vi "basement tank 2.vi"() -> ()   [LabVIEW 2019]
uses:
  <vilib>/NI/Current Value Table/Type Defs/Single Tag.ctl
  <vilib>/NI/Current Value Table/Type Defs/Data Types.ctl
  <vilib>/NI/STM/TCP/Read Meta Data (TCP Ref).vi
  <vilib>/NI/STM/TCP/Get Connection Reference (TCP).vi
  <vilib>/NI/AMC/Read Termination Message.vi
  <vilib>/NI/AMC/Create Single Message.vi
  <vilib>/NI/AMC/Update Message Routing Info.vi
  <vilib>/NI/STM/TCP/Read Meta Data (TCP Clst).vi
  <vilib>/NI/AMC/Globals.vi
  <vilib>/NI/STM/TCP/Write Message (TCP).vi
  <vilib>/NI/AMC/Send Message.vi
  <vilib>/NI/AMC/AMC.lvlib
  <vilib>/NI/STM/NI STM.lvlib
  <vilib>/NI/Current Value Table/Current Value Table.lvlib
panel:
  in  "Auto Level Main Tank":dbl(knob)=250.0 min=250.0 max=950.0 step=1.0 scale=200.0..1000.0 scale format="%#.3g"
  in  "Enable DI Auto Top-up":bool
  in  "CuOAddAmount":dbl caption="CuO grams to add" min=-1000.0 max=1000.0 step=1.0
  out "Grams CuO to Add":dbl format="%.1f"
  in  "Dose Extra Oxide":bool
  in  "Sulfuric Proc 2":dbl=2.0 caption="ml Acid Proc 2" min=0.0 max=5000.0 step=1.0
  in  "Trig Sulfuric Proc2":bool caption="Trigger Dose"
  out "Flow":bool
  in  "LEV Proc 2":dbl=2.0 caption="ml Lev Proc 2" min=0.0 max=1000.0 step=1.0
  in  "Trig Level Proc 2":bool caption="Trigger Dose"
  in  "UCON Proc 2":dbl=2.0 caption="ml UCON Proc 2" min=0.0 max=1000.0 step=1.0
  in  "Trig UCON Proc 2":bool caption="Trigger Dose"
  in  "SPS Proc 2":dbl=2.0 caption="ml SPS Proc 2" min=0.0 max=1000.0 step=1.0
  in  "Trig SPS Proc 2":bool caption="Trigger Dose"
  in  "BasT2_L Last Hr":bool
  in  "FlowInd OxSys":dbl(slide) scale=0.0..15.0
  in  "Supply Pressure (kPa)":dbl(knob)=50.0 min=50.0 max=200.0 step=5.0 scale=50.0..200.0
  in  "BasT2_P Last Hr":bool
  in  "BasT2_Flow Last Hr":bool
  out "Boiler Water Facilities Valve":dbl(slide) scale=0.0..100.0
  out "Tempered Water Facilities Valve":dbl(slide) scale=0.0..100.0
  out "Chilled Water Facilities Valve":dbl(slide) scale=0.0..100.0
  out "Total Flow (when operated with plating tanks)":dbl(knob) scale=0.0..150.0
  out "To Plating Process 3 & 4":bool
  out "ThreewayLowerElbow":bool
  out "PipeToTank":bool
  out "Tnk1Tee 2":bool
  out "PipeToPump 2":bool
  out "BTnk1 SG":dbl format="%.3f"
  in  "Specific Gravity":dbl(knob)=1.0 min=1.0 max=1.25 step=0.0025 scale=1.0..1.25
  out "OxideToFilter":bool
  out "Oxide Pump":bool
  out "Boolean 4":bool
  out "OxideDose Indicate":bool
  in  "Flow rate To Oxide":dbl(knob) scale=2.0..10.0
  in  "Oxide Dosing Enable":bool
  out "Chilled Injection":u8(slide) scale=0.0..100.0
  out "Tempered Injection":dbl(slide) scale=0.0..100.0
  in  "BasT3_T Last Hr":bool
  in  "Enable T-Control":bool
  in  "Temperature Setpoint":dbl(knob) step=0.1 scale=12.0..30.0 scale format="%#.1g"
  out "Boiler Water Out":dbl(knob) scale=10.0..110.0
  out "Boiler Water In":dbl(knob) scale=10.0..110.0
  out "Tempered Water Out":dbl(knob) scale=10.0..35.0
  out "Tempered Water In":dbl(knob) scale=10.0..35.0
  out "Chilled Water Out":dbl(knob) scale=0.0..25.0
  out "Chilled Water In":dbl(knob) scale=0.0..25.0
  in  "Tab Control":enum32{"Main Pump", "Lift Pump"}(tab)
  out "Amps":dbl format="%#.2g"
  out "Volts":dbl format="%#.1f"
  out "VFD T":dbl format="%#.2g"
  out "RPM":dbl format="%#.2f"
  out "Fault Code":dbl format="%#.2g"
  out "Freq":dbl format="%#.2g"
  out "Fault Code Ox Pmp":dbl caption="Fault Code" format="%#.2g"
  out "VFD T Ox Pmp":dbl caption="VFD T" format="%#.2g"
  out "Amps Ox Pmp":dbl caption="Amps" format="%#.2g"
  out "Volts Ox Pmp":dbl caption="Volts" format="%#.1f"
  out "Boolean 6":bool
  out "Circulator":bool
  out "HeatExchanger":bool
  out "Main Pump":bool
  out "Supply Pressure (kPa)":dbl(knob) scale=0.0..250.0
  out "Total Added":dbl format="%.2g"
  out "DI Flow (L/min)":dbl(knob) scale=0.0..100.0
  in  "Liters DI to Add":dbl(knob) min=0.0 max=500.0 step=1.0 scale=0.0..500.0
  in  "Add DI Water":bool
  in  "Drain System to Tree":bool
  in  "Enable Main Pump":bool
  out "E Stop":bool
  out "Run Enabled?":bool
  out "Supply Temperature":dbl(slide) scale=0.0..100.0
  out "Tank":dbl(slide) scale=0.0..1000.0
  in  "Machine":bool
  in  "Basement 4":bool
  in  "Dryer":bool
  in  "Rinse 4":bool
  in  "Rinse 3":bool
  in  "Rinse 2":bool
  in  "Basement 3":bool
  in  "Basement 2":bool
  in  "Basement 1":bool
  in  "Plater 6":bool
  in  "Plater 5":bool
  in  "Plater 4":bool
  in  "Plater 3":bool
  in  "Plater 2":bool
  in  "Plater 1":bool
  in  "Predip":bool
  in  "Rinse 1":bool
  in  "Cleaner":bool
  in  "Etch":bool
  out "status":string
  out "Tnk1Tee":bool
  out "PipeToPump":bool
  # "Module Selection"
  # "@"
  # "SG"
  # "L/min"
  # "Dosing"
  # "SPS"
  # "UCON"
  # "Leveler"
  # "Sulfuric Acid"
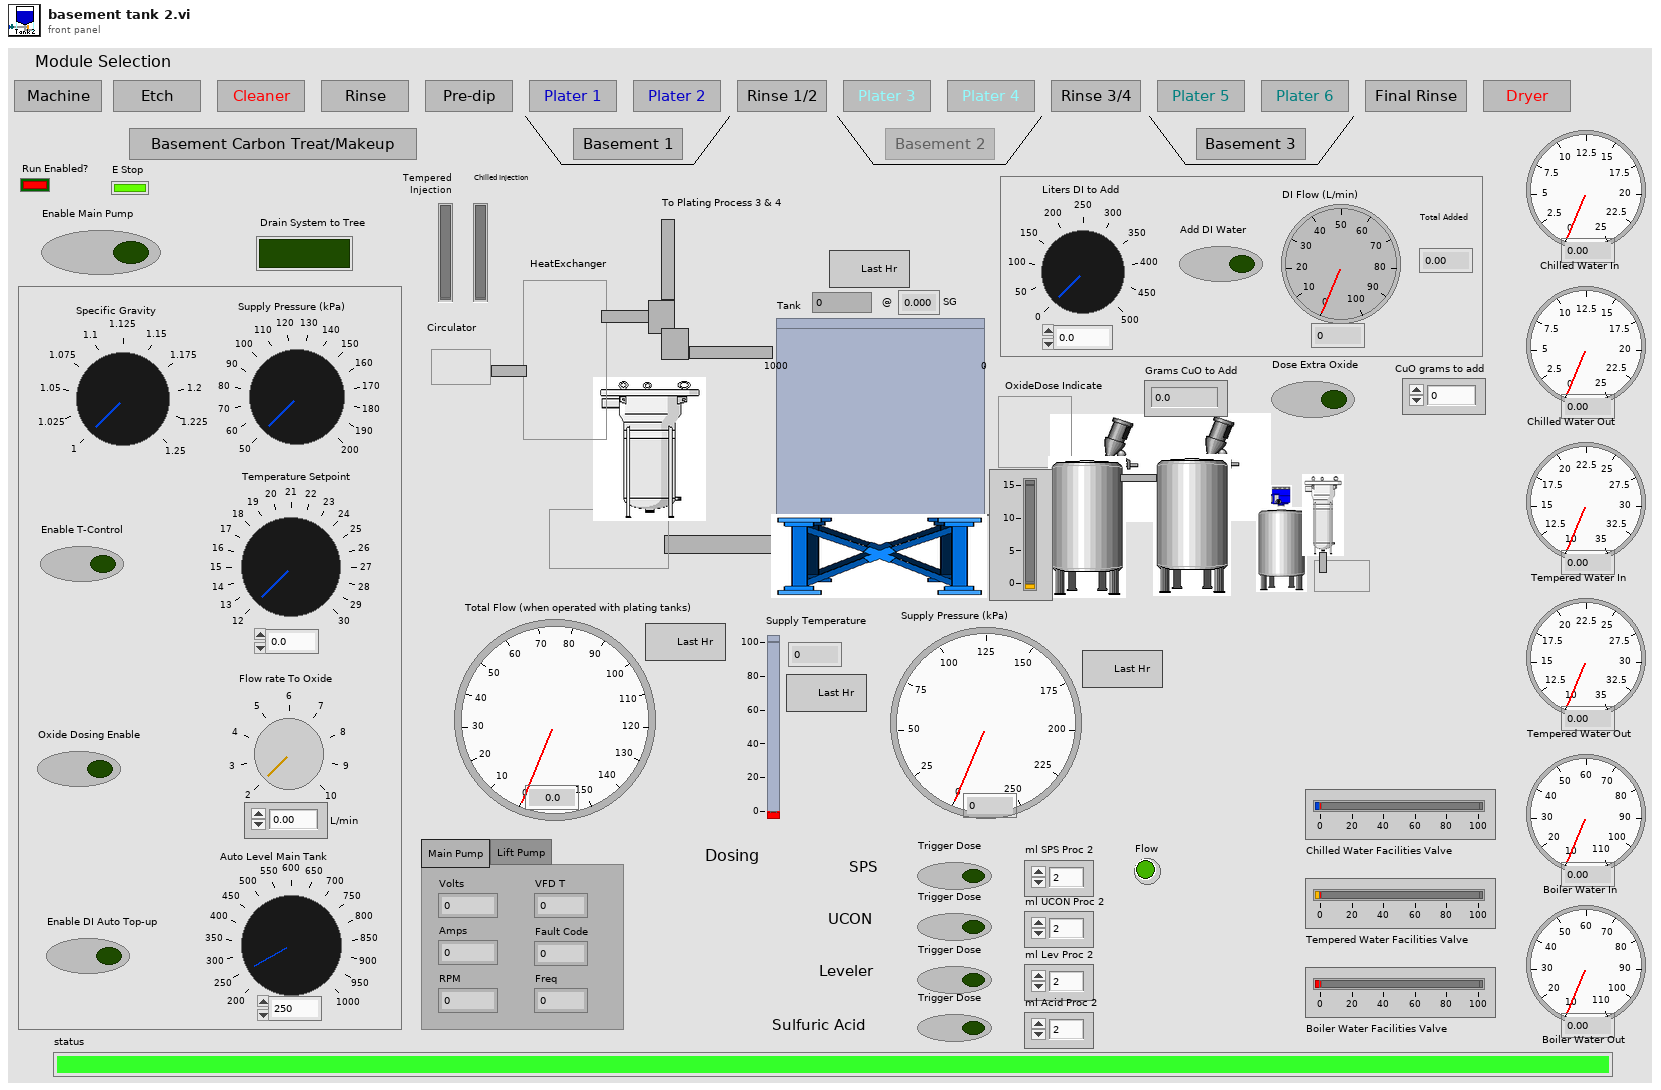
[diagram p1: front panel]
types:
  T1 = typedef "Current Value Table.lvlib/Single Tag.ctl" = cluster{"Data Type":T2, "Name":string, "Value":string, "Description":string}
  T2 = typedef "Current Value Table.lvlib/Data Types.ctl" = enum16{"Double", "Single", "I64", "I32", "I16", "I8", "U64", "U32", "U16", "U8", "String", "Boolean", "Array of U8", "Array of U16", "Array of U32", "Array of U64", "Array of I64", "Array of I32", "Array of I16", "Array of I8", "Array of Double", "Array of Single", "Array of Boolean", "Array of String"}
  T3 = typedef "NI STM.lvlib/TCP Connection Info.ctl" = cluster{"connection ID":refnum<k5>, "meta data":T4[]}
  T4 = typedef "NI STM.lvlib/MetaDataElement.ctl" = string
  T5 = typedef "AMC.lvlib/Message Queue.ctl" = refnum<queue>
  T6 = cluster{"Shift":bool, "Ctrl":bool, "Alt":bool, "Cmd":bool, "Opt":bool}
  T7 = enum8{"Enabled", "Disabled", "Disabled and Grayed Out"}
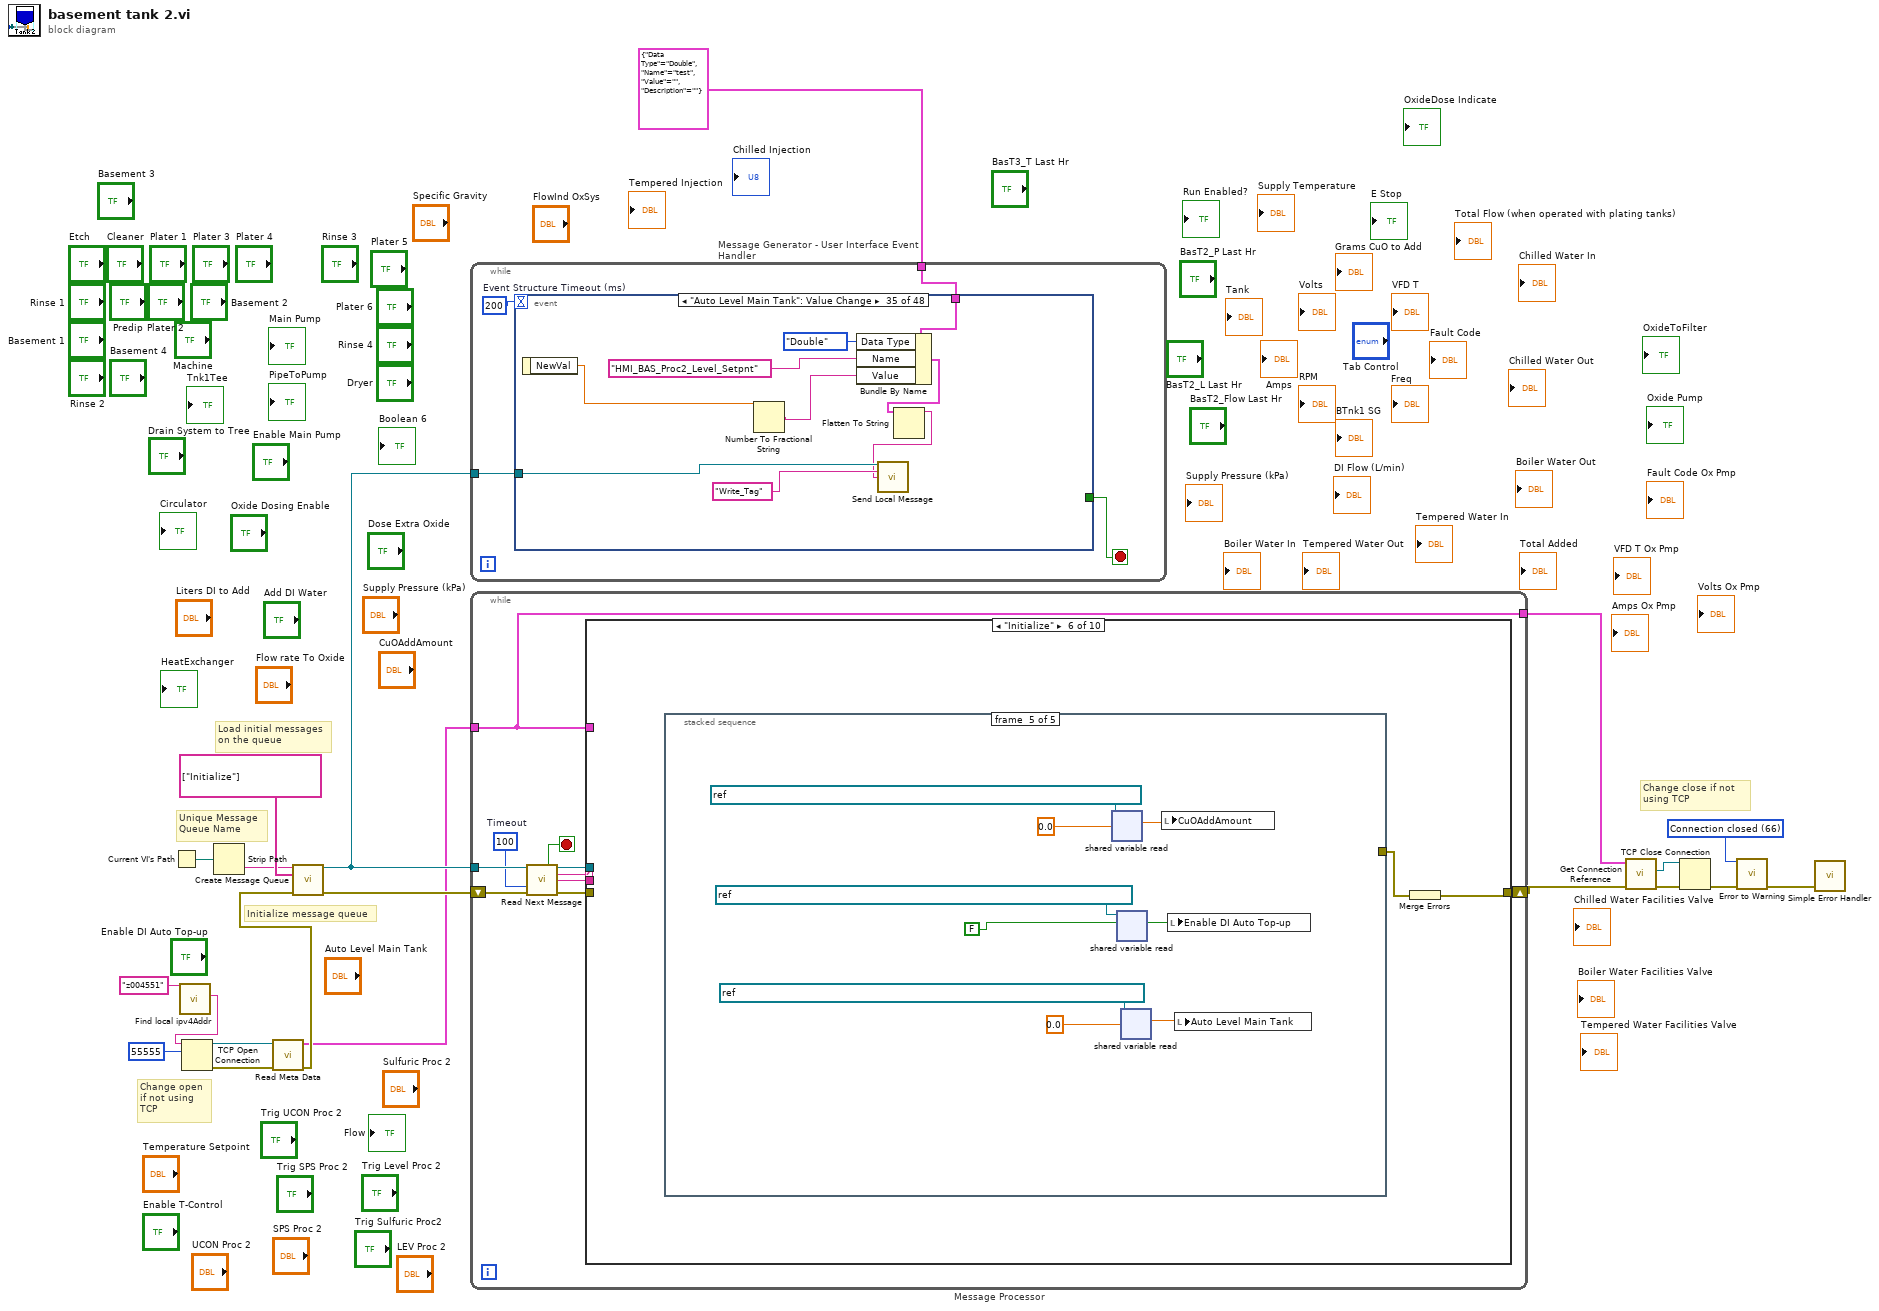
[diagram p0: block diagram]
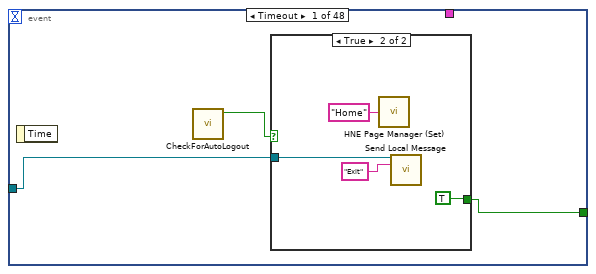
[diagram p2: hidden frame]
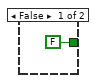
[diagram p3: hidden frame]
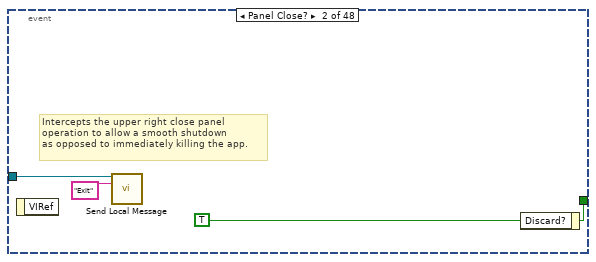
[diagram p4: hidden frame]
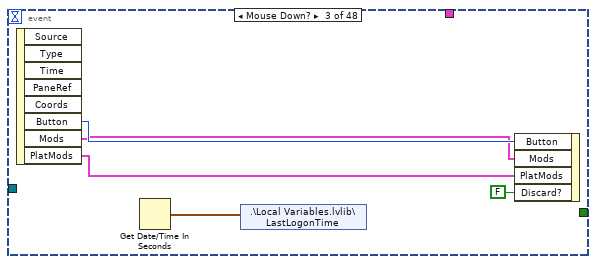
[diagram p5: hidden frame]
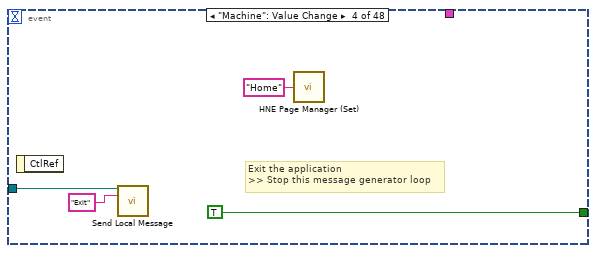
[diagram p6: hidden frame]
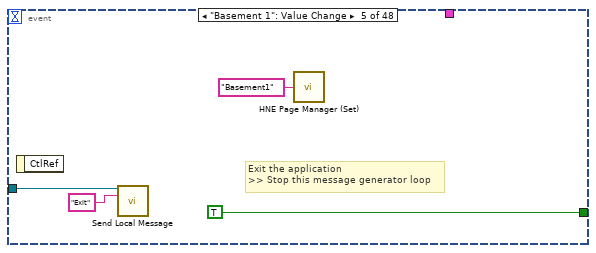
[diagram p7: hidden frame]
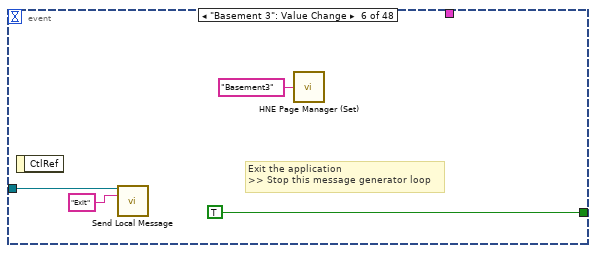
[diagram p8: hidden frame]
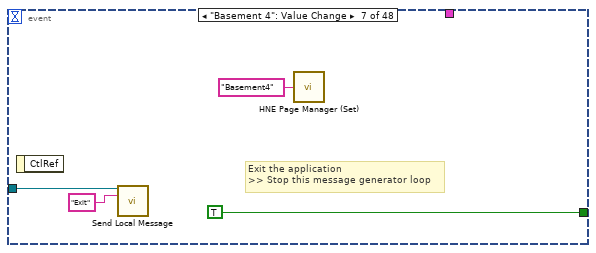
[diagram p9: hidden frame]
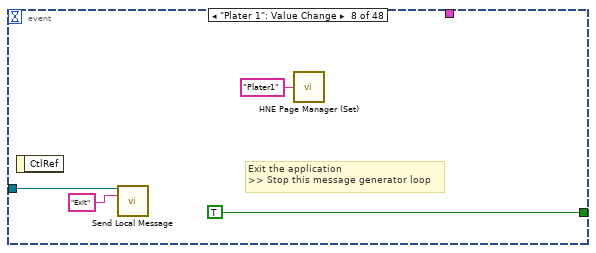
[diagram p10: hidden frame]
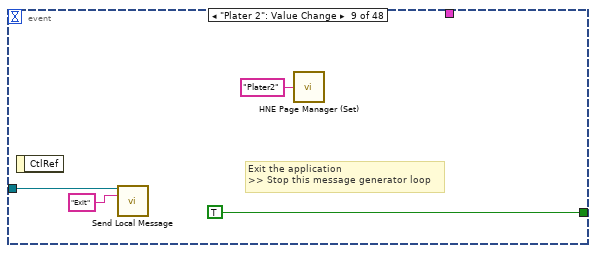
[diagram p11: hidden frame]
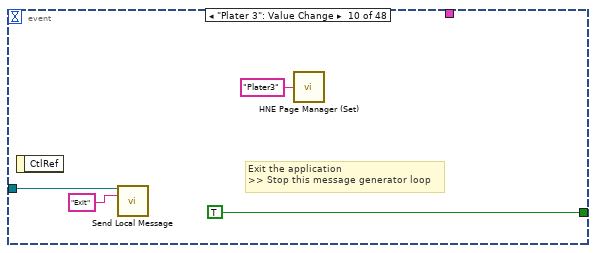
[diagram p12: hidden frame]
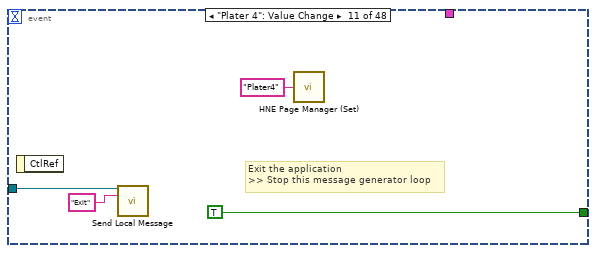
[diagram p13: hidden frame]
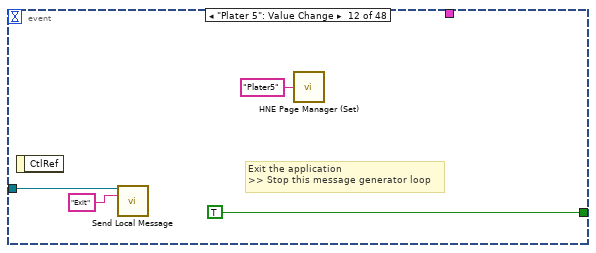
[diagram p14: hidden frame]
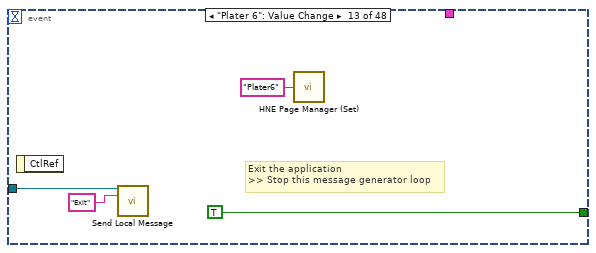
[diagram p15: hidden frame]
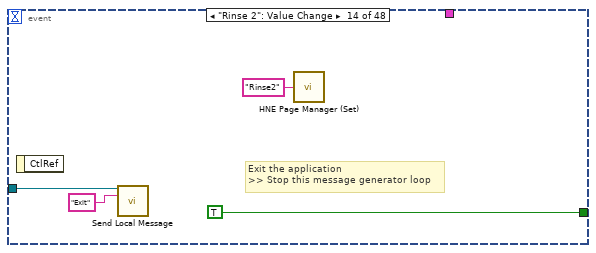
[diagram p16: hidden frame]
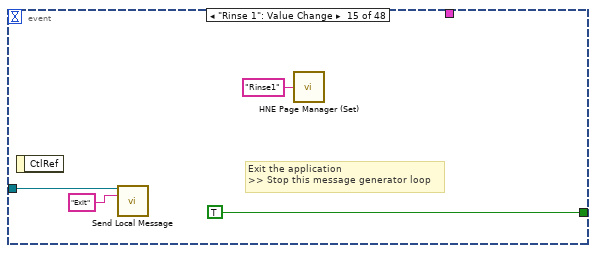
[diagram p17: hidden frame]
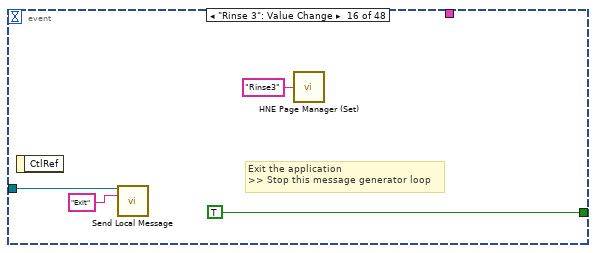
[diagram p18: hidden frame]
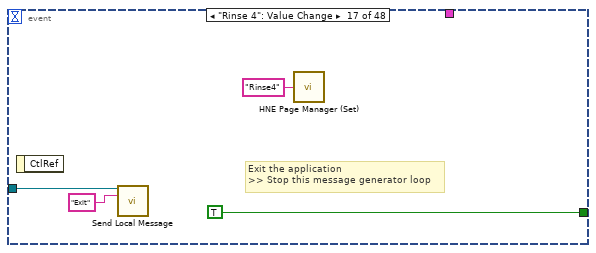
[diagram p19: hidden frame]
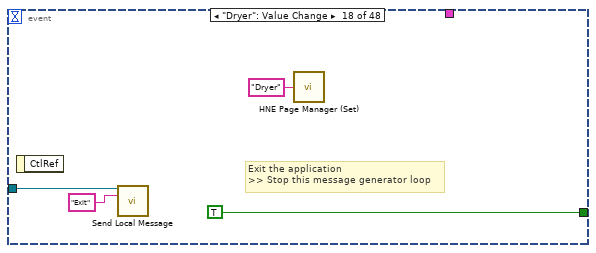
[diagram p20: hidden frame]
diagram:
  w9 = 66 items=["No Error", "Argument Error", "Memory Full", "Out of Zone", "End of File", "File Already Open", "Generic File IO Error", "File Not Found", "File Permission Error", "Disk Full", "Duplicate Path", "Too Many Files Open", "Not Enabled", "Resource File Not Found", "Cannot Add Resource", "Resource Not Found", "Image Not Found", "Image Memory Error", "Pen Does Not Exist", "Config Bad Type", "Config Token Not Found", "Config Parse Error", "Config Memory Error", "Bad External Code Format", "Bad External Code Offset", "External Code Not Present", "Null Window", "Destroy Window Mixup", "Null Menu", "Print Aborted", "Bad Print Record", "Print Driver Error", "Windows Error During Print", "Memory Error During Print", "Print Dialog Error", "Generic Print Error", "Invalid Device Refnum", "Device Not Found", "Device Parameter Error", "Device Unit Error", "Can't Open Device", "Device Call Aborted", "Generic Error", "Cancelled By User", "Object ID Too Low", "Object ID Too High", "Object Not In Heap", "Unknown Heap", "Bad DefProc ID", "DefProc Not In Table", "Message Out Of Range", "Null Method", "Unknown Message", "Manager Call Not Supported", "Bad address", "Connection In progress", "Connection timed out", "Connection is already in progress", "Network attribute not supported", "Network error", "Address in use", "System out of memory", "Connection aborted", "Connection refused", "Connection is not connected", "Connection is already connected", "Connection closed", "Initialize error (interapplication manager)", "Bad occurrence", "Wait on unbound occurrence handler", "Occurrence queue overflow", "Bad path", "Semaphore not signaled", "Unrecognized type (interapplication manager)"] ("1st Error to Convert")
  # "Change close if not using TCP"
  # "Change open if not using TCP"
  # "Initialize message queue"
  # "Unique Message\nQueue Name"
  # "Load initial messages\non the queue"
  n1 = Current VI's Path() -> (path=w16:path)
  n2 = call "Find local ipv4Addr.vi"("MachineToFind"="z004551" ("Target IP Address")) -> ("name"=w1:string)  [unwired: 9 in, 1 out]
  n3 = TCP Open Connection(address=w1, remote port or service name=u16 55555 ("remote port")) -> (connection ID=w14:refnum<k5>, error out=w13:errorcluster)  [unwired: 1 in, 2 out]
  n4 = Strip Path(path=w16) -> (name=w19:string)  [unwired: 1 out]
  n5 = call-poly <vilib>:"Read Meta Data.vi"("error in"=w13, "connection ID"=w14) -> ("error out"=w12:errorcluster, "connection info out"=w11:T3)  [unwired: 7 in, 1 out]
  n6 = call <vilib>:"Create Message Queue.vi"("message queue name"=w19, "initial message names"=string[] ["Initialize"], "error in"=w12) -> ("message queue out"=w18:T5, "error out"=w17:errorcluster)  [unwired: 11 in]
  n7 = while "Message Generator - User Interface Event Handler" {
    tunnel: w18 -> [w22]
    tunnel: T1 {"Data Type"=enum."Double", "Name"="test", "Value"="", "Description"=""} ("Tag") -> [w21]
    stop <- w23 stop-if-true
    w24 = 200  # Event Structure Timeout (ms)
    n8 = event shown="[34] \"Auto Level Main Tank\": Value Change" {
      selector: _ -> [_ _ _ _ _ _ _ _ _ _ _ _ _ _ _ _ _ _ _ _ _ _ _ _ _ _ _ _ _ _ _ _ _ _ _ _ _ _ _ _ _ _ _ _ _ _ _ _]
      dyn-events: _ -> [_ _ _ _ _ _ _ _ _ _ _ _ _ _ _ _ _ _ _ _ _ _ _ _ _ _ _ _ _ _ _ _ _ _ _ _ _ _ _ _ _ _ _ _ _ _ _ _]
      timeout: w24 -> [_ _ _ _ _ _ _ _ _ _ _ _ _ _ _ _ _ _ _ _ _ _ _ _ _ _ _ _ _ _ _ _ _ _ _ _ _ _ _ _ _ _ _ _ _ _ _ _]
      tunnel: [w25 w35 _ TRUE ("Discard?") TRUE ("Discard?") TRUE ("Discard?") TRUE ("Discard?") TRUE ("Discard?") TRUE ("Discard?") TRUE ("Discard?") TRUE ("Discard?") TRUE ("Discard?") TRUE ("Discard?") TRUE ("Discard?") TRUE ("Discard?") TRUE ("Discard?") TRUE ("Discard?") TRUE ("Discard?") TRUE ("Discard?") TRUE ("Discard?") TRUE ("Discard?") _ _ _ _ _ _ _ _ _ _ _ _ _ _ _ _ _ _ _ _ _ _ _ _ _ _ _] -> w23
      tunnel: w22 -> [w26 w33 _ w42 w46 w50 w54 w58 w62 w66 w70 w74 w78 w82 w86 w90 w94 w98 w102 w106 w110 w113 w124 w134 w144 w154 w164 w174 w184 w194 w204 w214 w224 w233 w242 w251 w260 w269 w278 w287 w296 w305 w314 w323 w324 w329 w334 w339]
      tunnel: w21 -> [_ _ _ _ _ _ _ _ _ _ _ _ _ _ _ _ _ _ _ _ _ _ w118 w128 w138 w148 w158 w168 w178 w188 w198 w208 w218 w229 w238 w247 w256 w265 w274 w283 w292 w301 w310 w319 _ _ _ _]
      event Timeout {
        n9 = event-data() -> ()  [unwired: 2 out]
        n10 = call "CheckForAutoLogout.vi"() -> ("Boolean"=w27:bool)  [unwired: 11 in]
        n11 = case shown="True" w27 {
          tunnel: [FALSE ("Discard?") TRUE ("Discard?")] -> w25
          tunnel: w26 -> [_ w29]
          frame False {
          }
          frame True {
            n12 = call <userlib>:"HNE Page Manager (Set).vi"("Next Page"="Home") -> ()  [unwired: 4 in, 1 out]
            n13 = call <vilib>:"Send Local Message.vi"("message queue in"=w29, "message name"="Exit") -> ()  [unwired: 11 in, 3 out]
          }
        }
      }
      event Panel Close? {
        w35 = TRUE ("Discard?")
        # "Intercepts the upper right close panel\noperation to allow a smooth shutdown\nas opposed to immediately killing the app."
        n14 = event-data() -> ()  [unwired: 2 out]
        n15 = call <vilib>:"Send Local Message.vi"("message queue in"=w33, "message name"="Exit") -> ()  [unwired: 11 in, 3 out]
        n16 = event-data("Discard?"=w35) -> ()  [unwired: 1 in, 1 out]
      }
      event Mouse Down? {
        n17 = event-data() -> ("Button"=w40:u16, "Mods"=w39:cluster{"Double Click":bool, "Menu Key":bool}, "PlatMods"=w38:T6)  [unwired: 6 out]
        n18 = Get Date/Time In Seconds() -> (seconds since 1Jan1904=w36:timestamp)
        n19 = shared-variable ".\\Local Variables.lvlib\\LastLogonTime"(w36) -> ()  [unwired: 1 in, 1 out]
        n20 = event-data("Button"=w40, "Mods"=w39, "PlatMods"=w38, "Discard?"=FALSE) -> ()  [unwired: 1 in, 1 out]
      }
      event "Machine": Value Change {
        # "Exit the application\n>> Stop this message generator loop"
        n21 = event-data() -> ()  [unwired: 2 out]
        n22 = call <vilib>:"Send Local Message.vi"("message queue in"=w42, "message name"="Exit") -> ()  [unwired: 11 in, 3 out]
        n23 = call <userlib>:"HNE Page Manager (Set).vi"("Next Page"="Home") -> ()  [unwired: 4 in, 1 out]
      }
      event "Basement 1": Value Change {
        # "Exit the application\n>> Stop this message generator loop"
        n24 = event-data() -> ()  [unwired: 2 out]
        n25 = call <vilib>:"Send Local Message.vi"("message queue in"=w46, "message name"="Exit") -> ()  [unwired: 11 in, 3 out]
        n26 = call <userlib>:"HNE Page Manager (Set).vi"("Next Page"="Basement1") -> ()  [unwired: 4 in, 1 out]
      }
      event "Basement 3": Value Change {
        # "Exit the application\n>> Stop this message generator loop"
        n27 = event-data() -> ()  [unwired: 2 out]
        n28 = call <vilib>:"Send Local Message.vi"("message queue in"=w50, "message name"="Exit") -> ()  [unwired: 11 in, 3 out]
        n29 = call <userlib>:"HNE Page Manager (Set).vi"("Next Page"="Basement3") -> ()  [unwired: 4 in, 1 out]
      }
      event "Basement 4": Value Change {
        # "Exit the application\n>> Stop this message generator loop"
        n30 = event-data() -> ()  [unwired: 2 out]
        n31 = call <vilib>:"Send Local Message.vi"("message queue in"=w54, "message name"="Exit") -> ()  [unwired: 11 in, 3 out]
        n32 = call <userlib>:"HNE Page Manager (Set).vi"("Next Page"="Basement4") -> ()  [unwired: 4 in, 1 out]
      }
      event "Plater 1": Value Change {
        # "Exit the application\n>> Stop this message generator loop"
        n33 = event-data() -> ()  [unwired: 2 out]
        n34 = call <vilib>:"Send Local Message.vi"("message queue in"=w58, "message name"="Exit") -> ()  [unwired: 11 in, 3 out]
        n35 = call <userlib>:"HNE Page Manager (Set).vi"("Next Page"="Plater1") -> ()  [unwired: 4 in, 1 out]
      }
      event "Plater 2": Value Change {
        # "Exit the application\n>> Stop this message generator loop"
        n36 = event-data() -> ()  [unwired: 2 out]
        n37 = call <vilib>:"Send Local Message.vi"("message queue in"=w62, "message name"="Exit") -> ()  [unwired: 11 in, 3 out]
        n38 = call <userlib>:"HNE Page Manager (Set).vi"("Next Page"="Plater2") -> ()  [unwired: 4 in, 1 out]
      }
      event "Plater 3": Value Change {
        # "Exit the application\n>> Stop this message generator loop"
        n39 = event-data() -> ()  [unwired: 2 out]
        n40 = call <vilib>:"Send Local Message.vi"("message queue in"=w66, "message name"="Exit") -> ()  [unwired: 11 in, 3 out]
        n41 = call <userlib>:"HNE Page Manager (Set).vi"("Next Page"="Plater3") -> ()  [unwired: 4 in, 1 out]
      }
      event "Plater 4": Value Change {
        # "Exit the application\n>> Stop this message generator loop"
        n42 = event-data() -> ()  [unwired: 2 out]
        n43 = call <vilib>:"Send Local Message.vi"("message queue in"=w70, "message name"="Exit") -> ()  [unwired: 11 in, 3 out]
        n44 = call <userlib>:"HNE Page Manager (Set).vi"("Next Page"="Plater4") -> ()  [unwired: 4 in, 1 out]
      }
      event "Plater 5": Value Change {
        # "Exit the application\n>> Stop this message generator loop"
        n45 = event-data() -> ()  [unwired: 2 out]
        n46 = call <vilib>:"Send Local Message.vi"("message queue in"=w74, "message name"="Exit") -> ()  [unwired: 11 in, 3 out]
        n47 = call <userlib>:"HNE Page Manager (Set).vi"("Next Page"="Plater5") -> ()  [unwired: 4 in, 1 out]
      }
      event "Plater 6": Value Change {
        # "Exit the application\n>> Stop this message generator loop"
        n48 = event-data() -> ()  [unwired: 2 out]
        n49 = call <vilib>:"Send Local Message.vi"("message queue in"=w78, "message name"="Exit") -> ()  [unwired: 11 in, 3 out]
        n50 = call <userlib>:"HNE Page Manager (Set).vi"("Next Page"="Plater6") -> ()  [unwired: 4 in, 1 out]
      }
      event "Rinse 2": Value Change {
        # "Exit the application\n>> Stop this message generator loop"
        n51 = event-data() -> ()  [unwired: 2 out]
        n52 = call <vilib>:"Send Local Message.vi"("message queue in"=w82, "message name"="Exit") -> ()  [unwired: 11 in, 3 out]
        n53 = call <userlib>:"HNE Page Manager (Set).vi"("Next Page"="Rinse2") -> ()  [unwired: 4 in, 1 out]
      }
      event "Rinse 1": Value Change {
        # "Exit the application\n>> Stop this message generator loop"
        n54 = event-data() -> ()  [unwired: 2 out]
        n55 = call <vilib>:"Send Local Message.vi"("message queue in"=w86, "message name"="Exit") -> ()  [unwired: 11 in, 3 out]
        n56 = call <userlib>:"HNE Page Manager (Set).vi"("Next Page"="Rinse1") -> ()  [unwired: 4 in, 1 out]
      }
      event "Rinse 3": Value Change {
        # "Exit the application\n>> Stop this message generator loop"
        n57 = event-data() -> ()  [unwired: 2 out]
        n58 = call <vilib>:"Send Local Message.vi"("message queue in"=w90, "message name"="Exit") -> ()  [unwired: 11 in, 3 out]
        n59 = call <userlib>:"HNE Page Manager (Set).vi"("Next Page"="Rinse3") -> ()  [unwired: 4 in, 1 out]
      }
      event "Rinse 4": Value Change {
        # "Exit the application\n>> Stop this message generator loop"
        n60 = event-data() -> ()  [unwired: 2 out]
        n61 = call <vilib>:"Send Local Message.vi"("message queue in"=w94, "message name"="Exit") -> ()  [unwired: 11 in, 3 out]
        n62 = call <userlib>:"HNE Page Manager (Set).vi"("Next Page"="Rinse4") -> ()  [unwired: 4 in, 1 out]
      }
      event "Dryer": Value Change {
        # "Exit the application\n>> Stop this message generator loop"
        n63 = event-data() -> ()  [unwired: 2 out]
        n64 = call <vilib>:"Send Local Message.vi"("message queue in"=w98, "message name"="Exit") -> ()  [unwired: 11 in, 3 out]
        n65 = call <userlib>:"HNE Page Manager (Set).vi"("Next Page"="Dryer") -> ()  [unwired: 4 in, 1 out]
      }
      event "Predip": Value Change {
        # "Exit the application\n>> Stop this message generator loop"
        n66 = event-data() -> ()  [unwired: 2 out]
        n67 = call <vilib>:"Send Local Message.vi"("message queue in"=w102, "message name"="Exit") -> ()  [unwired: 11 in, 3 out]
        n68 = call <userlib>:"HNE Page Manager (Set).vi"("Next Page"="Predip") -> ()  [unwired: 4 in, 1 out]
      }
      event "Cleaner": Value Change {
        # "Exit the application\n>> Stop this message generator loop"
        n69 = event-data() -> ()  [unwired: 2 out]
        n70 = call <vilib>:"Send Local Message.vi"("message queue in"=w106, "message name"="Exit") -> ()  [unwired: 11 in, 3 out]
        n71 = call <userlib>:"HNE Page Manager (Set).vi"("Next Page"="Clean") -> ()  [unwired: 4 in, 1 out]
      }
      event "Etch": Value Change {
        # "Exit the application\n>> Stop this message generator loop"
        n72 = event-data() -> ()  [unwired: 2 out]
        n73 = call <vilib>:"Send Local Message.vi"("message queue in"=w110, "message name"="Exit") -> ()  [unwired: 11 in, 3 out]
        n74 = call <userlib>:"HNE Page Manager (Set).vi"("Next Page"="Etch") -> ()  [unwired: 4 in, 1 out]
      }
      event Menu Selection (User) {
        # "Add run-time menu items to the message\nqueue. The message handler case names must match the menu ItemTag names."
        n75 = event-data() -> ("ItemTag"=w114:string)  [unwired: 1 out]
        n76 = call <vilib>:"Send Local Message.vi"("message queue in"=w113, "message name"=w114) -> ()  [unwired: 11 in, 3 out]
      }
      event "Enable Main Pump": Value Change {
        n77 = event-data() -> ("NewVal"=w117:bool)  [unwired: 1 out]
        n78 = Boolean To (0,1)(Boolean=w117) -> (0, 1=w123:i16)
        n79 = Number To Decimal String(number=w123) -> (decimal integer string=w122:string)  [unwired: 1 in]
        n80 = Bundle By Name(cluster=w118, "Data Type"=Data_Types."Boolean", "Name"="HMI_Enable_BTnk2_Pump", "Value"=w122) -> (w121:T1)
        n81 = Flatten To String(anything=w121) -> (data string=w115:string)  [unwired: 3 in, 2 out]
        n82 = call <vilib>:"Send Local Message.vi"("message queue in"=w124, "message name"="Write_Tag", "message value"=w115) -> ()  [unwired: 10 in, 3 out]
      }
      event "Drain System to Tree": Value Change {
        n83 = event-data() -> ("NewVal"=w127:bool)  [unwired: 1 out]
        n84 = Boolean To (0,1)(Boolean=w127) -> (0, 1=w133:i16)
        n85 = Number To Decimal String(number=w133) -> (decimal integer string=w132:string)  [unwired: 1 in]
        n86 = Bundle By Name(cluster=w128, "Data Type"=Data_Types."Boolean", "Name"="HMI_Drain_BTank2", "Value"=w132) -> (w131:T1)
        n87 = Flatten To String(anything=w131) -> (data string=w125:string)  [unwired: 3 in, 2 out]
        n88 = call <vilib>:"Send Local Message.vi"("message queue in"=w134, "message name"="Write_Tag", "message value"=w125) -> ()  [unwired: 10 in, 3 out]
      }
      event "Enable T-Control": Value Change {
        n89 = event-data() -> ("NewVal"=w137:bool)  [unwired: 1 out]
        n90 = Boolean To (0,1)(Boolean=w137) -> (0, 1=w143:i16)
        n91 = Number To Decimal String(number=w143) -> (decimal integer string=w142:string)  [unwired: 1 in]
        n92 = Bundle By Name(cluster=w138, "Data Type"=Data_Types."Boolean", "Name"="HMI_BAS_Tank2_TControl_Enable", "Value"=w142) -> (w141:T1)
        n93 = Flatten To String(anything=w141) -> (data string=w135:string)  [unwired: 3 in, 2 out]
        n94 = call <vilib>:"Send Local Message.vi"("message queue in"=w144, "message name"="Write_Tag", "message value"=w135) -> ()  [unwired: 10 in, 3 out]
      }
      event "Oxide Dosing Enable": Value Change {
        n95 = event-data() -> ("NewVal"=w147:bool)  [unwired: 1 out]
        n96 = Boolean To (0,1)(Boolean=w147) -> (0, 1=w153:i16)
        n97 = Number To Decimal String(number=w153) -> (decimal integer string=w152:string)  [unwired: 1 in]
        n98 = Bundle By Name(cluster=w148, "Data Type"=Data_Types."Boolean", "Name"="HMI_Proc2_Run_OxideSys", "Value"=w152) -> (w151:T1)
        n99 = Flatten To String(anything=w151) -> (data string=w145:string)  [unwired: 3 in, 2 out]
        n100 = call <vilib>:"Send Local Message.vi"("message queue in"=w154, "message name"="Write_Tag", "message value"=w145) -> ()  [unwired: 10 in, 3 out]
      }
      event "Trig SPS Proc 2": Value Change {
        n101 = event-data() -> ("NewVal"=w157:bool)  [unwired: 1 out]
        n102 = Boolean To (0,1)(Boolean=w157) -> (0, 1=w163:i16)
        n103 = Number To Decimal String(number=w163) -> (decimal integer string=w162:string)  [unwired: 1 in]
        n104 = Bundle By Name(cluster=w158, "Data Type"=Data_Types."Boolean", "Name"="HMI_Dose_SPS_Proc2", "Value"=w162) -> (w161:T1)
        n105 = Flatten To String(anything=w161) -> (data string=w155:string)  [unwired: 3 in, 2 out]
        n106 = call <vilib>:"Send Local Message.vi"("message queue in"=w164, "message name"="Write_Tag", "message value"=w155) -> ()  [unwired: 10 in, 3 out]
      }
      event "Trig UCON Proc 2": Value Change {
        n107 = event-data() -> ("NewVal"=w167:bool)  [unwired: 1 out]
        n108 = Boolean To (0,1)(Boolean=w167) -> (0, 1=w173:i16)
        n109 = Number To Decimal String(number=w173) -> (decimal integer string=w172:string)  [unwired: 1 in]
        n110 = Bundle By Name(cluster=w168, "Data Type"=Data_Types."Boolean", "Name"="HMI_Dose_UCON_Proc2", "Value"=w172) -> (w171:T1)
        n111 = Flatten To String(anything=w171) -> (data string=w165:string)  [unwired: 3 in, 2 out]
        n112 = call <vilib>:"Send Local Message.vi"("message queue in"=w174, "message name"="Write_Tag", "message value"=w165) -> ()  [unwired: 10 in, 3 out]
      }
      event "Trig Level Proc 2": Value Change {
        n113 = event-data() -> ("NewVal"=w177:bool)  [unwired: 1 out]
        n114 = Boolean To (0,1)(Boolean=w177) -> (0, 1=w183:i16)
        n115 = Number To Decimal String(number=w183) -> (decimal integer string=w182:string)  [unwired: 1 in]
        n116 = Bundle By Name(cluster=w178, "Data Type"=Data_Types."Boolean", "Name"="HMI_Dose_Leveler_Proc2", "Value"=w182) -> (w181:T1)
        n117 = Flatten To String(anything=w181) -> (data string=w175:string)  [unwired: 3 in, 2 out]
        n118 = call <vilib>:"Send Local Message.vi"("message queue in"=w184, "message name"="Write_Tag", "message value"=w175) -> ()  [unwired: 10 in, 3 out]
      }
      event "Trig Sulfuric Proc2": Value Change {
        n119 = event-data() -> ("NewVal"=w187:bool)  [unwired: 1 out]
        n120 = Boolean To (0,1)(Boolean=w187) -> (0, 1=w193:i16)
        n121 = Number To Decimal String(number=w193) -> (decimal integer string=w192:string)  [unwired: 1 in]
        n122 = Bundle By Name(cluster=w188, "Data Type"=Data_Types."Boolean", "Name"="HMI_Dose_Acid_Proc2", "Value"=w192) -> (w191:T1)
        n123 = Flatten To String(anything=w191) -> (data string=w185:string)  [unwired: 3 in, 2 out]
        n124 = call <vilib>:"Send Local Message.vi"("message queue in"=w194, "message name"="Write_Tag", "message value"=w185) -> ()  [unwired: 10 in, 3 out]
      }
      event "Add DI Water": Value Change {
        n125 = event-data() -> ("NewVal"=w197:bool)  [unwired: 1 out]
        n126 = Boolean To (0,1)(Boolean=w197) -> (0, 1=w203:i16)
        n127 = Number To Decimal String(number=w203) -> (decimal integer string=w202:string)  [unwired: 1 in]
        n128 = Bundle By Name(cluster=w198, "Data Type"=Data_Types."Boolean", "Name"="HMI_BAS_Proc2_AddDIVolume", "Value"=w202) -> (w201:T1)
        n129 = Flatten To String(anything=w201) -> (data string=w195:string)  [unwired: 3 in, 2 out]
        n130 = call <vilib>:"Send Local Message.vi"("message queue in"=w204, "message name"="Write_Tag", "message value"=w195) -> ()  [unwired: 10 in, 3 out]
      }
      event "Enable DI Auto Top-up": Value Change {
        n131 = event-data() -> ("NewVal"=w207:bool)  [unwired: 1 out]
        n132 = Boolean To (0,1)(Boolean=w207) -> (0, 1=w213:i16)
        n133 = Number To Decimal String(number=w213) -> (decimal integer string=w212:string)  [unwired: 1 in]
        n134 = Bundle By Name(cluster=w208, "Data Type"=Data_Types."Boolean", "Name"="HMI_BAS_Proc2_Level_Auto", "Value"=w212) -> (w211:T1)
        n135 = Flatten To String(anything=w211) -> (data string=w205:string)  [unwired: 3 in, 2 out]
        n136 = call <vilib>:"Send Local Message.vi"("message queue in"=w214, "message name"="Write_Tag", "message value"=w205) -> ()  [unwired: 10 in, 3 out]
      }
      event "Dose Extra Oxide": Value Change {
        n137 = event-data() -> ("NewVal"=w217:bool)  [unwired: 1 out]
        n138 = Boolean To (0,1)(Boolean=w217) -> (0, 1=w223:i16)
        n139 = Number To Decimal String(number=w223) -> (decimal integer string=w222:string)  [unwired: 1 in]
        n140 = Bundle By Name(cluster=w218, "Data Type"=Data_Types."Boolean", "Name"="HMI_Proc2_Add_CuOxide", "Value"=w222) -> (w221:T1)
        n141 = Flatten To String(anything=w221) -> (data string=w215:string)  [unwired: 3 in, 2 out]
        n142 = call <vilib>:"Send Local Message.vi"("message queue in"=w224, "message name"="Write_Tag", "message value"=w215) -> ()  [unwired: 10 in, 3 out]
      }
      event "Liters DI to Add": Value Change {
        n143 = event-data() -> ("NewVal"=w226:dbl)  [unwired: 1 out]
        n144 = Number To Fractional String(number=w226) -> (F-format string=w225:string)  [unwired: 3 in]
        n145 = Bundle By Name(cluster=w229, "Data Type"=Data_Types."Double", "Name"="HMI_BAS_Proc2_DI_Setpnt", "Value"=w225) -> (w232:T1)
        n146 = Flatten To String(anything=w232) -> (data string=w227:string)  [unwired: 3 in, 2 out]
        n147 = call <vilib>:"Send Local Message.vi"("message queue in"=w233, "message name"="Write_Tag", "message value"=w227) -> ()  [unwired: 10 in, 3 out]
      }
      event "Auto Level Main Tank": Value Change {
        n148 = event-data() -> ("NewVal"=w235:dbl)  [unwired: 1 out]
        n149 = Number To Fractional String(number=w235) -> (F-format string=w234:string)  [unwired: 3 in]
        n150 = Bundle By Name(cluster=w238, "Data Type"=Data_Types."Double", "Name"="HMI_BAS_Proc2_Level_Setpnt", "Value"=w234) -> (w241:T1)
        n151 = Flatten To String(anything=w241) -> (data string=w236:string)  [unwired: 3 in, 2 out]
        n152 = call <vilib>:"Send Local Message.vi"("message queue in"=w242, "message name"="Write_Tag", "message value"=w236) -> ()  [unwired: 10 in, 3 out]
      }
      event "Temperature Setpoint": Value Change {
        n153 = event-data() -> ("NewVal"=w244:dbl)  [unwired: 1 out]
        n154 = Number To Fractional String(number=w244) -> (F-format string=w243:string)  [unwired: 3 in]
        n155 = Bundle By Name(cluster=w247, "Data Type"=Data_Types."Double", "Name"="HMI_BAS_TNK2_T_Setpoint", "Value"=w243) -> (w250:T1)
        n156 = Flatten To String(anything=w250) -> (data string=w245:string)  [unwired: 3 in, 2 out]
        n157 = call <vilib>:"Send Local Message.vi"("message queue in"=w251, "message name"="Write_Tag", "message value"=w245) -> ()  [unwired: 10 in, 3 out]
      }
      event "Flow rate To Oxide": Value Change {
        n158 = event-data() -> ("NewVal"=w253:dbl)  [unwired: 1 out]
        n159 = Number To Fractional String(number=w253) -> (F-format string=w252:string)  [unwired: 3 in]
        n160 = Bundle By Name(cluster=w256, "Data Type"=Data_Types."Double", "Name"="HMI_Proc2_OxFlow_SetPnt", "Value"=w252) -> (w259:T1)
        n161 = Flatten To String(anything=w259) -> (data string=w254:string)  [unwired: 3 in, 2 out]
        n162 = call <vilib>:"Send Local Message.vi"("message queue in"=w260, "message name"="Write_Tag", "message value"=w254) -> ()  [unwired: 10 in, 3 out]
      }
      event "Specific Gravity": Value Change {
        n163 = event-data() -> ("NewVal"=w262:dbl)  [unwired: 1 out]
        n164 = Number To Fractional String(number=w262) -> (F-format string=w261:string)  [unwired: 3 in]
        n165 = Bundle By Name(cluster=w265, "Data Type"=Data_Types."Double", "Name"="HMI_BAS_Proc2_Tank_SG", "Value"=w261) -> (w268:T1)
        n166 = Flatten To String(anything=w268) -> (data string=w263:string)  [unwired: 3 in, 2 out]
        n167 = call <vilib>:"Send Local Message.vi"("message queue in"=w269, "message name"="Write_Tag", "message value"=w263) -> ()  [unwired: 10 in, 3 out]
      }
      event "Supply Pressure (kPa)": Value Change {
        n168 = event-data() -> ("NewVal"=w271:dbl)  [unwired: 1 out]
        n169 = Number To Fractional String(number=w271) -> (F-format string=w270:string)  [unwired: 3 in]
        n170 = Bundle By Name(cluster=w274, "Data Type"=Data_Types."Double", "Name"="HMI_BAS_TNK2_P_Setpoint", "Value"=w270) -> (w277:T1)
        n171 = Flatten To String(anything=w277) -> (data string=w272:string)  [unwired: 3 in, 2 out]
        n172 = call <vilib>:"Send Local Message.vi"("message queue in"=w278, "message name"="Write_Tag", "message value"=w272) -> ()  [unwired: 10 in, 3 out]
      }
      event "SPS Proc 2": Value Change {
        n173 = event-data() -> ("NewVal"=w280:dbl)  [unwired: 1 out]
        n174 = Number To Fractional String(number=w280) -> (F-format string=w279:string)  [unwired: 3 in]
        n175 = Bundle By Name(cluster=w283, "Data Type"=Data_Types."Double", "Name"="HMI_SPS_Amount_Proc2", "Value"=w279) -> (w286:T1)
        n176 = Flatten To String(anything=w286) -> (data string=w281:string)  [unwired: 3 in, 2 out]
        n177 = call <vilib>:"Send Local Message.vi"("message queue in"=w287, "message name"="Write_Tag", "message value"=w281) -> ()  [unwired: 10 in, 3 out]
      }
      event "UCON Proc 2": Value Change {
        n178 = event-data() -> ("NewVal"=w289:dbl)  [unwired: 1 out]
        n179 = Number To Fractional String(number=w289) -> (F-format string=w288:string)  [unwired: 3 in]
        n180 = Bundle By Name(cluster=w292, "Data Type"=Data_Types."Double", "Name"="HMI_UCON_Amount_Proc2", "Value"=w288) -> (w295:T1)
        n181 = Flatten To String(anything=w295) -> (data string=w290:string)  [unwired: 3 in, 2 out]
        n182 = call <vilib>:"Send Local Message.vi"("message queue in"=w296, "message name"="Write_Tag", "message value"=w290) -> ()  [unwired: 10 in, 3 out]
      }
      event "LEV Proc 2": Value Change {
        n183 = event-data() -> ("NewVal"=w298:dbl)  [unwired: 1 out]
        n184 = Number To Fractional String(number=w298) -> (F-format string=w297:string)  [unwired: 3 in]
        n185 = Bundle By Name(cluster=w301, "Data Type"=Data_Types."Double", "Name"="HMI_Leveler_Amount_Proc2", "Value"=w297) -> (w304:T1)
        n186 = Flatten To String(anything=w304) -> (data string=w299:string)  [unwired: 3 in, 2 out]
        n187 = call <vilib>:"Send Local Message.vi"("message queue in"=w305, "message name"="Write_Tag", "message value"=w299) -> ()  [unwired: 10 in, 3 out]
      }
      event "Sulfuric Proc 2": Value Change {
        n188 = event-data() -> ("NewVal"=w307:dbl)  [unwired: 1 out]
        n189 = Number To Fractional String(number=w307) -> (F-format string=w306:string)  [unwired: 3 in]
        n190 = Bundle By Name(cluster=w310, "Data Type"=Data_Types."Double", "Name"="HMI_Acid_Amount_Proc2", "Value"=w306) -> (w313:T1)
        n191 = Flatten To String(anything=w313) -> (data string=w308:string)  [unwired: 3 in, 2 out]
        n192 = call <vilib>:"Send Local Message.vi"("message queue in"=w314, "message name"="Write_Tag", "message value"=w308) -> ()  [unwired: 10 in, 3 out]
      }
      event "CuOAddAmount": Value Change {
        n193 = event-data() -> ("NewVal"=w316:dbl)  [unwired: 1 out]
        n194 = Number To Fractional String(number=w316) -> (F-format string=w315:string)  [unwired: 3 in]
        n195 = Bundle By Name(cluster=w319, "Data Type"=Data_Types."Double", "Name"="HMI_Proc2_CuOxideAddAmnt", "Value"=w315) -> (w322:T1)
        n196 = Flatten To String(anything=w322) -> (data string=w317:string)  [unwired: 3 in, 2 out]
        n197 = call <vilib>:"Send Local Message.vi"("message queue in"=w323, "message name"="Write_Tag", "message value"=w317) -> ()  [unwired: 10 in, 3 out]
      }
      event "BasT3_T Last Hr": Value Change {
        n198 = event-data() -> ("NewVal"=w325:bool)  [unwired: 6 out]
        n199 = case shown="True" w325 {
          tunnel: w324 -> [_ w328]
          frame False {
          }
          frame True {
            n200 = call <vilib>:"Send Local Message.vi"("message queue in"=w328, "message name"="DisplayLastHr", "message value"="BAS_Proc2_T") -> ()  [unwired: 10 in, 3 out]
          }
        }
      }
      event "BasT2_Flow Last Hr": Value Change {
        n201 = event-data() -> ("NewVal"=w330:bool)  [unwired: 6 out]
        n202 = case shown="True" w330 {
          tunnel: w329 -> [_ w333]
          frame False {
          }
          frame True {
            n203 = call <vilib>:"Send Local Message.vi"("message queue in"=w333, "message name"="DisplayLastHr", "message value"="BAS_Proc2_Total_Flow") -> ()  [unwired: 10 in, 3 out]
          }
        }
      }
      event "BasT2_P Last Hr": Value Change {
        n204 = event-data() -> ("NewVal"=w335:bool)  [unwired: 6 out]
        n205 = case shown="True" w335 {
          tunnel: w334 -> [_ w338]
          frame False {
          }
          frame True {
            n206 = call <vilib>:"Send Local Message.vi"("message queue in"=w338, "message name"="DisplayLastHr", "message value"="BAS_Proc2_P") -> ()  [unwired: 10 in, 3 out]
          }
        }
      }
      event "BasT2_L Last Hr": Value Change {
        n207 = event-data() -> ("NewVal"=w340:bool)  [unwired: 6 out]
        n208 = case shown="True" w340 {
          tunnel: w339 -> [_ w343]
          frame False {
          }
          frame True {
            n209 = call <vilib>:"Send Local Message.vi"("message queue in"=w343, "message name"="DisplayLastHr", "message value"="BAS_Proc2_Tank_Level") -> ()  [unwired: 10 in, 3 out]
          }
        }
      }
    }
  }
  n210 = while "Message Processor" {
    shift-left: w17 -> [w349]
    shift-right: [w353] -> w4
    tunnel: w18 -> [w350]
    tunnel: w11 -> [w344]
    tunnel: [w344] -> w5
    stop <- w352 stop-if-true
    w345 = 100  # Timeout
    n211 = call <vilib>:"Read Next Message.vi"("message queue in"=w350, "timeout (1 ms)"=w345, "error in"=w349) -> ("exit process?"=w352:bool, "message queue out"=w351:T5, "message name"=w347:string, "message value"=w346:string, "error out"=w348:errorcluster)  [unwired: 5 in, 3 out]
    n212 = case shown="\"Initialize\"" w347 {
      selector: w347 -> [_ _ w428 _ _ _ _ _ _ _]
      tunnel: w351 -> [_ _ _ _ _ _ w497 _ _ _]
      tunnel: w348 -> [w354 _ w429 w430 w432 _ w498 w500 w502 w506]
      tunnel: [w354 w356 w429 errorcluster {"status"=FALSE, "code"=0, "source"=""} ("error out") w432 w433 w496 w500 w501 w506] -> w353
      tunnel: w346 -> [_ _ _ _ _ _ _ _ w503 w507]
      tunnel: w344 -> [_ _ _ _ _ _ _ _ w505 _]
      frame "---------- Framework Operations ----------" {
        # "Dummy case to add a seperator in the Case Structure menu"
      }
      frame "", "Idle" {
        n213 = stacked-sequence {
          tunnel: [w367 _ _ _] -> w355
          frame #0 {
            n214 = shared-variable-read(refnum<k21> "ni.var.psp://z004551/CDL0100 ReadWriteTags/HMI_Drain_BTank2" ("shared variable refnum in"), FALSE) -> (w361:errorcluster, w364:bool)  [unwired: 1 in, 2 out]
            n215 = shared-variable-read(refnum<k21> "ni.var.psp://z004551/CDL0100 ReadWriteTags/HMI_BAS_Proc2_AddDIVolume" ("shared variable refnum in"), FALSE) -> (w368:errorcluster, w371:bool)  [unwired: 1 in, 2 out]
            n216 = shared-variable-read(refnum<k21> "ni.var.psp://z004551/CDL0100 ReadWriteTags/HMI_Enable_BTnk2_Pump" ("shared variable refnum in"), FALSE) -> (w369:errorcluster, w360:bool)  [unwired: 1 in, 2 out]
            n217 = control-ref of="Enable Main Pump"() -> (w362:refnum<vi>)
            n218 = case shown="True" w364 {
              tunnel: [T7."Enabled" ("Disabled") T7."Disabled and Grayed Out" ("Disabled")] -> w363
              frame False {
              }
              frame True {
              }
            }
            n219 = call <userlib>:"Boolean Trigger__ogtk.vi"("Boolean Input"=w371) -> ("Falling Edge"=w370:bool)  [unwired: 1 in, 1 out]
            n220 = call <userlib>:"Boolean Trigger__ogtk.vi"("Boolean Input"=w360) -> ("Rising Edge"=w358:bool, "Falling Edge"=w359:bool)  [unwired: 1 in]
            n221 = case shown="True" w358 {
              frame False {
              }
              frame True {
                n222 = local write "Enable Main Pump"(TRUE) -> ()
              }
            }
            n223 = case shown="True" w359 {
              frame False {
              }
              frame True {
                n224 = local write "Enable Main Pump"(FALSE) -> ()
              }
            }
            n225 = case shown="True" w370 {
              frame False {
              }
              frame True {
                n226 = local write "Add DI Water"(FALSE) -> ()
              }
            }
            n227 = property class="Bool (strict)"(reference=w362, "DisabledEnum"=w363) -> ()  [unwired: 1 in, 2 out]
            n228 = Merge Errors(w369, w368, w361) -> (w367:errorcluster)
          }
          frame #1 {
            n229 = shared-variable-read(refnum<k21> "ni.var.psp://z004551/CDL0100 ReadTags/IO_Bas_Tnk2_3Way_At_Recirc" ("shared variable refnum in"), FALSE) -> (w384:bool)  [unwired: 1 in, 3 out]
            n230 = shared-variable-read(refnum<k21> "ni.var.psp://z004551/CDL0100 ReadTags/IO_Bas_Tnk2_3Way_At_Open" ("shared variable refnum in"), FALSE) -> (w386:bool)  [unwired: 1 in, 3 out]
            n231 = shared-variable-read(refnum<k21> "ni.var.psp://z004551/CDL0100 ReadTags/IO_Bas_Tnk2_3Way_At_Closed" ("shared variable refnum in"), FALSE) -> (w388:bool)  [unwired: 1 in, 3 out]
            n232 = Or(x=w386, y=w384) -> (x .or. y?=→"PipeToTank" →"ThreewayLowerElbow":bool)
            n233 = Or(x=w388, y=w386) -> (x .or. y?=w381:bool)
            "To Plating Process 3 & 4" <- w381
            n234 = Or(x=w381, y=w384) -> (x .or. y?=→"Tnk1Tee 2" →"PipeToPump 2":bool)
          }
          frame #2 {
            n235 = control-ref of="Trig Sulfuric Proc2"() -> (w403:refnum<vi>)
            n236 = control-ref of="Trig SPS Proc 2"() -> (w398:refnum<vi>)
            n237 = shared-variable-read(refnum<k21> "ni.var.psp://z004551/CDL0100 ReadTags/BAS_Proc2_Oxide_FlowRate" ("shared variable refnum in"), 0.0) -> (w395:dbl)  [unwired: 1 in, 3 out]
            n238 = shared-variable-read(refnum<k21> "ni.var.psp://z004551/CDL0100 ReadWriteTags/HMI_Dose_SPS_Proc2" ("shared variable refnum in"), FALSE) -> (w400:bool)  [unwired: 1 in, 3 out]
            n239 = shared-variable-read(refnum<k21> "ni.var.psp://z004551/CDL0100 ReadWriteTags/HMI_Dose_Acid_Proc2" ("shared variable refnum in"), FALSE) -> (w405:bool)  [unwired: 1 in, 3 out]
            n240 = Greater?(x=w395, y=1.0) -> (0:→"Boolean 4":bool)
            n241 = call <userlib>:"Boolean Trigger__ogtk.vi"("Boolean Input"=w400) -> ("Falling Edge"=w399:bool)  [unwired: 1 in, 1 out]
            n242 = call <userlib>:"Boolean Trigger__ogtk.vi"("Boolean Input"=w405) -> ("Falling Edge"=w404:bool)  [unwired: 1 in, 1 out]
            n243 = case shown="True" w404 {
              tunnel: w403 -> [_ w411]
              frame False {
              }
              frame True {
                n244 = property class="Bool (strict)"(reference=w411, "Value"=FALSE) -> ()  [unwired: 1 in, 2 out]
              }
            }
            n245 = case shown="True" w399 {
              tunnel: w398 -> [_ w409]
              frame False {
              }
              frame True {
                n246 = property class="Bool (strict)"(reference=w409, "Value"=FALSE) -> ()  [unwired: 1 in, 2 out]
              }
            }
          }
          frame #3 {
            n247 = control-ref of="Trig UCON Proc 2"() -> (w417:refnum<vi>)
            n248 = control-ref of="Trig Level Proc 2"() -> (w412:refnum<vi>)
            n249 = shared-variable-read(refnum<k21> "ni.var.psp://z004551/CDL0100 ReadWriteTags/HMI_Dose_UCON_Proc2" ("shared variable refnum in"), FALSE) -> (w419:bool)  [unwired: 1 in, 3 out]
            n250 = shared-variable-read(refnum<k21> "ni.var.psp://z004551/CDL0100 ReadWriteTags/HMI_Dose_Leveler_Proc2" ("shared variable refnum in"), FALSE) -> (w414:bool)  [unwired: 1 in, 3 out]
            n251 = call <userlib>:"Boolean Trigger__ogtk.vi"("Boolean Input"=w419) -> ("Falling Edge"=w418:bool)  [unwired: 1 in, 1 out]
            n252 = call <userlib>:"Boolean Trigger__ogtk.vi"("Boolean Input"=w414) -> ("Falling Edge"=w413:bool)  [unwired: 1 in, 1 out]
            n253 = case shown="True" w418 {
              tunnel: w417 -> [_ w424]
              frame False {
              }
              frame True {
                n254 = property class="Bool (strict)"(reference=w424, "Value"=FALSE) -> ()  [unwired: 1 in, 2 out]
              }
            }
            n255 = case shown="True" w413 {
              tunnel: w412 -> [_ w423]
              frame False {
              }
              frame True {
                n256 = property class="Bool (strict)"(reference=w423, "Value"=FALSE) -> ()  [unwired: 1 in, 2 out]
              }
            }
          }
        }
        n257 = control-ref of="status"() -> (w357:refnum<vi>)
        n258 = call <userlib>:"TAE Format Alarm Ticker.vi"("Alarm Ticker Ref"=w357) -> ()  [unwired: 15 in]
        n259 = Merge Errors(w355) -> (w356:errorcluster)
      }
      frame "Missing Message Handler", Default {
        # "Call this case if a message is received that is not handled \nby any other case. Typically this is a programming error\nas a result of a typo or unhandled message/missing message handler."
        n260 = Format Into String(format string="DevError: Missing message handler for '%s\" message." ("message"), w428) -> (resulting string=w426:string)  [unwired: 2 in, 1 out]
        n261 = One Button Dialog(message=w426) -> ()  [unwired: 2 out]
      }
      frame "Error" {
        # "General Error Case - this case is called if an error is passed using the error cluster below. Typically most new errors should be handed in each individual case and not passed in the rror cluster. If necessary a custom error handler case should be added and called from other cases."
        n262 = call <vilib>:"Simple Error Handler.vi"("error in (no error)"=w430) -> ()  [unwired: 1 in, 8 out]
      }
      frame "---------- Generic Operations ----------" {
        # "Dummy case to add a seperator in the Case Structure menu"
      }
      frame "Initialize" {
        n263 = stacked-sequence {
          tunnel: [w435 _ _ _ _] -> w434
          frame #0 {
            n264 = shared-variable-read(refnum<k21> "ni.var.psp://z004551/CDL0100 ReadWriteTags/HMI_BAS_Proc2_AddDIVolume" ("shared variable refnum in"), FALSE) -> (w439:bool)  [unwired: 1 in, 3 out]
            n265 = shared-variable-read(refnum<k21> "ni.var.psp://z004551/CDL0100 ReadWriteTags/HMI_Enable_BTnk2_Pump" ("shared variable refnum in"), FALSE) -> (w435:errorcluster, w445:bool)  [unwired: 1 in, 2 out]
            n266 = shared-variable-read(refnum<k21> "ni.var.psp://z004551/CDL0100 ReadWriteTags/HMI_BAS_Proc2_DI_Setpnt" ("shared variable refnum in"), 0.0) -> (w440:dbl)  [unwired: 1 in, 3 out]
            n267 = shared-variable-read(refnum<k21> "ni.var.psp://z004551/CDL0100 ReadWriteTags/HMI_BAS_Tank2_TControl_Enable" ("shared variable refnum in"), FALSE) -> (w436:bool)  [unwired: 1 in, 3 out]
            n268 = local write "Add DI Water"(w439) -> ()
            n269 = local write "Enable Main Pump"(w445) -> ()
            n270 = local write "Liters DI to Add"(w440) -> ()
            n271 = local write "Enable T-Control"(w436) -> ()
          }
          frame #1 {
            n272 = shared-variable-read(refnum<k21> "ni.var.psp://z004551/CDL0100 ReadWriteTags/HMI_BAS_TNK2_T_Setpoint" ("shared variable refnum in"), 0.0) -> (w460:dbl)  [unwired: 1 in, 3 out]
            n273 = shared-variable-read(refnum<k21> "ni.var.psp://z004551/CDL0100 ReadWriteTags/HMI_BAS_Proc2_Tank_SG" ("shared variable refnum in"), 1.0) -> (w451:dbl)  [unwired: 1 in, 3 out]
            n274 = shared-variable-read(refnum<k21> "ni.var.psp://z004551/CDL0100 ReadWriteTags/HMI_BAS_TNK2_P_Setpoint" ("shared variable refnum in"), 1.0) -> (w448:dbl)  [unwired: 1 in, 3 out]
            n275 = shared-variable-read(refnum<k21> "ni.var.psp://z004551/CDL0100 ReadWriteTags/HMI_Proc2_Run_OxideSys" ("shared variable refnum in"), FALSE) -> (w457:bool)  [unwired: 1 in, 3 out]
            n276 = shared-variable-read(refnum<k21> "ni.var.psp://z004551/CDL0100 ReadWriteTags/HMI_Proc2_OxFlow_SetPnt" ("shared variable refnum in"), 0.0) -> (w454:dbl)  [unwired: 1 in, 3 out]
            n277 = local write "Temperature Setpoint"(w460) -> ()
            n278 = local write "Oxide Dosing Enable"(w457) -> ()
            n279 = local write "Supply Pressure (kPa)"(w448) -> ()
            n280 = local write "Specific Gravity"(w451) -> ()
            n281 = local write "Flow rate To Oxide"(w454) -> ()
          }
          frame #2 {
            n282 = shared-variable-read(refnum<k21> "ni.var.psp://z004551/CDL0100 ReadWriteTags/HMI_Dose_SPS_Proc2" ("shared variable refnum in"), FALSE) -> (w466:bool)  [unwired: 1 in, 3 out]
            n283 = shared-variable-read(refnum<k21> "ni.var.psp://z004551/CDL0100 ReadWriteTags/HMI_UCON_Amount_Proc2" ("shared variable refnum in"), 0.0) -> (w463:dbl)  [unwired: 1 in, 3 out]
            n284 = shared-variable-read(refnum<k21> "ni.var.psp://z004551/CDL0100 ReadWriteTags/HMI_Dose_UCON_Proc2" ("shared variable refnum in"), FALSE) -> (w464:bool)  [unwired: 1 in, 3 out]
            n285 = shared-variable-read(refnum<k21> "ni.var.psp://z004551/CDL0100 ReadWriteTags/HMI_SPS_Amount_Proc2" ("shared variable refnum in"), 0.0) -> (w465:dbl)  [unwired: 1 in, 3 out]
            n286 = local write "Trig SPS Proc 2"(w466) -> ()
            n287 = local write "UCON Proc 2"(w463) -> ()
            n288 = local write "Trig UCON Proc 2"(w464) -> ()
            n289 = local write "SPS Proc 2"(w465) -> ()
          }
          frame #3 {
            n290 = shared-variable-read(refnum<k21> "ni.var.psp://z004551/CDL0100 ReadWriteTags/HMI_Leveler_Amount_Proc2" ("shared variable refnum in"), 0.0) -> (w477:dbl)  [unwired: 1 in, 3 out]
            n291 = shared-variable-read(refnum<k21> "ni.var.psp://z004551/CDL0100 ReadWriteTags/HMI_Dose_Leveler_Proc2" ("shared variable refnum in"), FALSE) -> (w478:bool)  [unwired: 1 in, 3 out]
            n292 = shared-variable-read(refnum<k21> "ni.var.psp://z004551/CDL0100 ReadWriteTags/HMI_Acid_Amount_Proc2" ("shared variable refnum in"), 0.0) -> (w476:dbl)  [unwired: 1 in, 3 out]
            n293 = shared-variable-read(refnum<k21> "ni.var.psp://z004551/CDL0100 ReadWriteTags/HMI_Dose_Acid_Proc2" ("shared variable refnum in"), FALSE) -> (w475:bool)  [unwired: 1 in, 3 out]
            n294 = local write "Trig Level Proc 2"(w478) -> ()
            n295 = local write "LEV Proc 2"(w477) -> ()
            n296 = local write "Sulfuric Proc 2"(w476) -> ()
            n297 = local write "Trig Sulfuric Proc2"(w475) -> ()
          }
          frame #4 {
            n298 = shared-variable-read(refnum<k21> "ni.var.psp://z004551/CDL0100 ReadWriteTags/HMI_Proc2_CuOxideAddAmnt" ("shared variable refnum in"), 0.0) -> (w493:dbl)  [unwired: 1 in, 3 out]
            n299 = shared-variable-read(refnum<k21> "ni.var.psp://z004551/CDL0100 ReadWriteTags/HMI_BAS_Proc2_Level_Auto" ("shared variable refnum in"), FALSE) -> (w490:bool)  [unwired: 1 in, 3 out]
            n300 = shared-variable-read(refnum<k21> "ni.var.psp://z004551/CDL0100 ReadWriteTags/HMI_BAS_Proc2_Level_Setpnt" ("shared variable refnum in"), 0.0) -> (w487:dbl)  [unwired: 1 in, 3 out]
            n301 = local write "CuOAddAmount"(w493) -> ()
            n302 = local write "Enable DI Auto Top-up"(w490) -> ()
            n303 = local write "Auto Level Main Tank"(w487) -> ()
          }
        }
        n304 = Merge Errors(w434) -> (w433:errorcluster)
      }
      frame "Exit" {
        # "Destroy message queue >> this will halt the UI event handler loop"
        # "Stop the VI\n>> Perform any cleanup tasks in this message case.\n>> Clear display before closing."
        n305 = call <vilib>:"Destroy Message Queue.vi"("message queue in"=w497, "error in"=w498) -> ("error out"=w496:errorcluster)  [unwired: 11 in, 2 out]
        n306 = local write "status"("" ("Status")) -> ()
      }
      frame "---------- Application Operations ----------" {
        # "Dummy case to add a seperator in the Case Structure menu"
      }
      frame "Write_Tag" {
        n307 = call-poly <vilib>:"Write Message.vi"("error in"=w502, "data"=w503, "name"="WriteTag", "connection info in"=w505) -> ("error out"=w501:errorcluster)  [unwired: 6 in, 1 out]
      }
      frame "DisplayLastHr" {
        n308 = call "Trace Variable 1 hour Popup.vi"("Tag"=w507) -> ()  [unwired: 11 in]
      }
    }
  }
  n309 = call-poly <vilib>:"Get Connection Reference.vi"("error in"=w4, "connection info in"=w5) -> ("error out"=w8:errorcluster, "connection ID out"=w7:refnum<k5>)  [unwired: 8 out]
  n310 = TCP Close Connection(connection ID=w7, error in (no error)=w8) -> (error out=w10:errorcluster)  [unwired: 2 out]
  n311 = call <vilib>:"Error to Warning.vi"("1st Error to Convert"=w9, "error in"=w10) -> ("warning out"=w6:errorcluster)  [unwired: 3 in, 10 out]
  n312 = call <vilib>:"Simple Error Handler.vi"("error in (no error)"=w6) -> ()  [unwired: 4 in, 5 out]
